vi "my글로벌.vi"() -> ()   [LabVIEW 2014]
panel:
  in  "data":dbl
  out "stop":bool
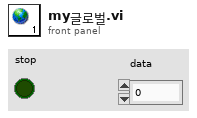
[diagram p1: front panel]
diagram:
